vi "Replace Array Subset (Value[]).vi"(5 "JSON Array":refnum<class "JSON Value.lvclass">, 7 "index":i32, 9 "new element/subarray":refnum<class "JSON Value.lvclass">[](array[class]), 11 "error in":errorcluster) -> (6 "output JSON Array":refnum<class "JSON Value.lvclass">, 15 "error out":errorcluster)   [LabVIEW 2016, in "JSON Value.lvclass"]
doc: "Replaces an element or subarray in an array at the point you specify in index."
uses:
  JSON Value.lvclass
  JSON Value.lvclass/JSON Value.ctl
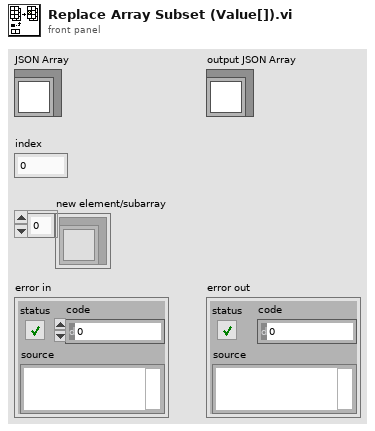
[diagram p1: front panel]
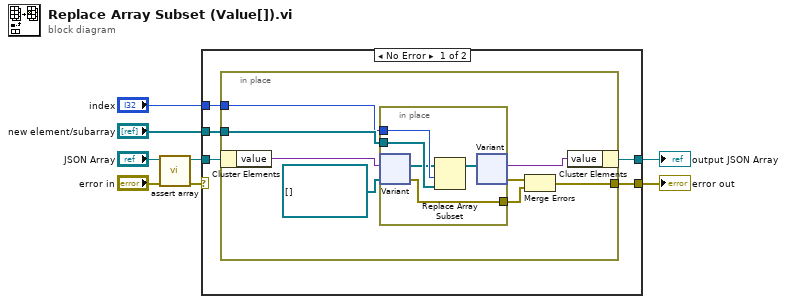
[diagram p0: block diagram]
diagram:
  n1 = call "assert array.vi"("error in (no error)"="error in", "JSON Value in"="JSON Array") -> ("error out"=w1:errorcluster, "JSON Value out"=w4:refnum<class "JSON Value.lvclass">)  [unwired: 8 in]
  n2 = case shown="No Error" w1 {
    selector: w1 -> [_ w27]
    tunnel: "index" -> [w13 _]
    tunnel: [w12 w28] -> w6
    tunnel: "new element/subarray" -> [w11 _]
    tunnel: w4 -> [w10 w28]
    tunnel: [w9 w27] -> w3
    frame No Error {
      n3 = in-place {
        in-place-border: w11 -> [w21]
        in-place-border: w13 -> [w20]
        in-place-border: [w14] -> w9
        n4 = in-place-cluster #1(w10) -> ("value"=w19:variant)
        n5 = in-place {
          in-place-border: w21 -> [w26]
          in-place-border: w20 -> [w25]
          in-place-border: [w22] -> w15
          n6 = in-place-variant #2(w19, refnum<class "JSON Value.lvclass">[] [] ("output array")) -> (w24:refnum<class "JSON Value.lvclass">[], w22:errorcluster)
          n7 = Replace Array Subset(array=w24, new element=w26, index=w25) -> (w23:refnum<class "JSON Value.lvclass">[])
          n8 = in-place-variant #2(w23) -> (w17:variant, w16:errorcluster)
        }
        n9 = Merge Errors(w16, w15) -> (w14:errorcluster)
        n10 = in-place-cluster #1("value"=w17) -> (w12:refnum<class "JSON Value.lvclass">)
      }
    }
    frame Error {
    }
  }
  "output JSON Array" <- w6
  "error out" <- w3
